vi "Message-handler.vi"(8 "error in (no error)":errorcluster, 11 "PD in":T1) -> (0 "error out":errorcluster, 3 "PD out":T1)   [LabVIEW 2013, in "SLMControl.lvlib" / "SC-Main.lvclass"]
doc: "Simple example of a continuous communication monitor loop.\nThe function continuously monitors the incomming (client) communication channel. At regular intervals, or after receiving a message, the client activity is reaffirmed through a 'heartbeat' message to the server.\nA new message is handled through the 'Process-received-message' function, which checks the message origins, determines the appropriate client action and executes this action."
uses:
  SC-Main.lvclass
  Object-reference.ctl
  SC-Main.lvclass/SC-Main.ctl
  Read Client.vi
  Client/Sources/SC-Client.lvclass
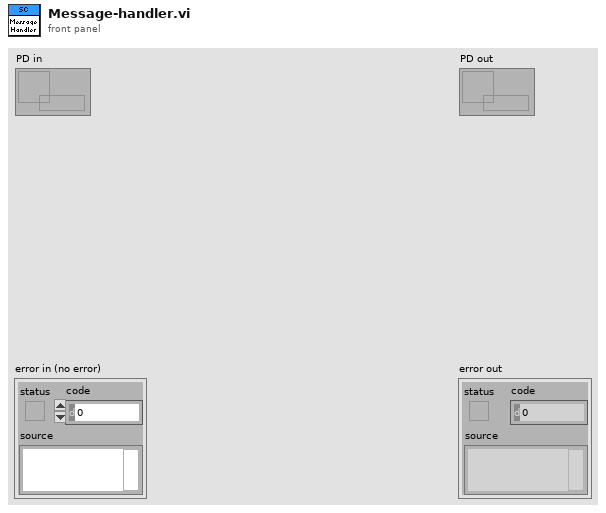
[diagram p1: front panel]
types:
  T1 = typedef "SLMControl.lvlib/SC-Main.lvclass/Object-reference.ctl" = refnum<data-value>
  T2 = typedef "SLMControl.lvlib/SC-Client.lvclass/Object-reference.ctl" = refnum<data-value>
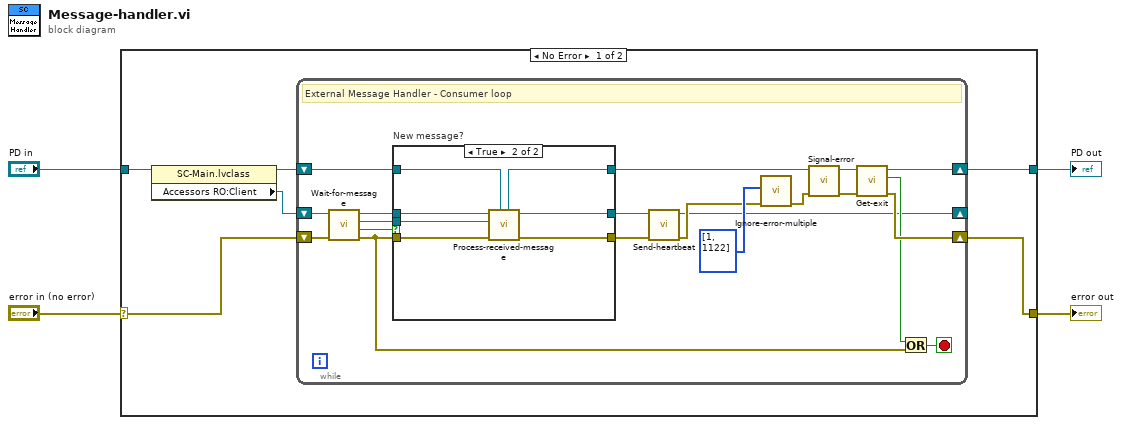
[diagram p0: block diagram]
diagram:
  n1 = case shown="No Error" "error in (no error)" {
    selector: "error in (no error)" -> [w10 w42]
    tunnel: [w5 w42] -> w3
    tunnel: [w6 w41] -> w1
    tunnel: "PD in" -> [w9 w41]
    frame No Error {
      n2 = property class="SC-Main.lvclass"(reference=w9) -> (reference out=w7:T1, "Accessors RO:Client"=w8:T2)  [unwired: 1 in, 1 out]
      n3 = while {
        shift-right: [w21] -> w5
        shift-left: w10 -> [w28]
        shift-right: [w11] -> _
        shift-left: w8 -> [w30]
        shift-right: [w22] -> w6
        shift-left: w7 -> [w23]
        stop <- w20 stop-if-true
        # "External Message Handler - Consumer loop"
        n4 = call "Wait-for-message.vi"("error in (no error)"=w28, "Client in"=w30) -> ("error out"=w18:errorcluster, "New message?"=w26:bool, "Message"=w27:refnum<class "Message.lvclass">, "Client out"=w29:T2)  [unwired: 6 in]
        n5 = case "New message?" shown="True" w26 {
          tunnel: w29 -> [w33 w40]
          tunnel: [w33 w39] -> w25
          tunnel: w18 -> [w32 w38]
          tunnel: w27 -> [_ w37]
          tunnel: [w32 w36] -> w24
          tunnel: w23 -> [w31 w35]
          tunnel: [w31 w34] -> w15
          frame False {
          }
          frame True {
            n6 = call "Process-received-message.vi"("Data ref in"=w35, "error in (no error)"=w38, "Message"=w37, "Client in"=w40) -> ("error out"=w36:errorcluster, "Client out"=w39:T2, "Data ref out"=w34:T1)  [unwired: 5 in]
          }
        }
        n7 = call "Send-heartbeat.vi"("error in (no error)"=w24, "Client in"=w25) -> ("error out"=w16:errorcluster, "Client out"=w11:T2)  [unwired: 8 in]
        n8 = call "Ignore-error-multiple.vi"("error in (no error)"=w16, "Errors to ignore (1)"=i32[] [1, 1122]) -> ("error out"=w12:errorcluster)  [unwired: 9 in]
        n9 = call "Signal-error.vi"("error in (no error)"=w12, "Data in"=w15) -> ("error out"=w13:errorcluster, "Data out"=w14:T1)  [unwired: 8 in]
        n10 = call "Get-exit.vi"("error in (no error)"=w13, "Object ref in"=w14) -> ("error out"=w21:errorcluster, "Exit?"=w19:bool, "Object ref out"=w22:T1)  [unwired: 7 in]
        n11 = Or(x=w19, y=w18) -> (x .or. y?=w20:bool)
      }
    }
    frame Error {
    }
  }
  "error out" <- w3
  "PD out" <- w1
